vi "NIIE_Get Icon Editor Source Paths.vi"() -> (0 "IconEditorSourcePaths":path[](array[path]))   [LabVIEW 2021]
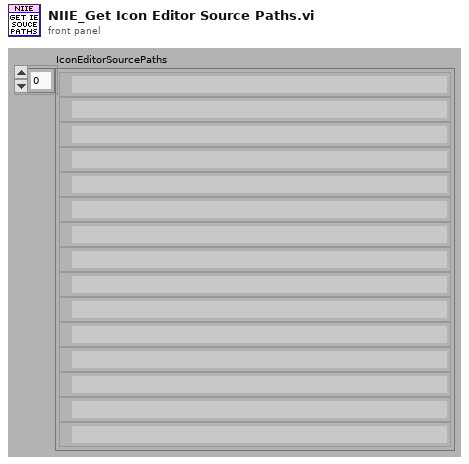
[diagram p1: front panel]
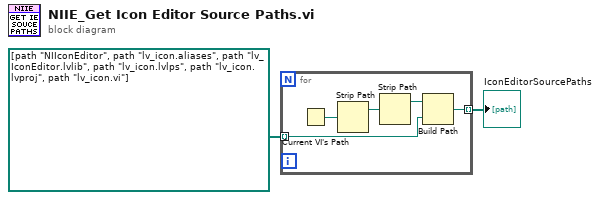
[diagram p0: block diagram]
diagram:
  n1 = for {
    tunnel: [w6] -> w2 mode=indexing
    tunnel: path[] [path "NIIconEditor", path "lv_icon.aliases", path "lv_IconEditor.lvlib", path "lv_icon.lvlps", path "lv_icon.lvproj", path "lv_icon.vi"] ("Array 2") -> [w5] mode=indexing
    n2 = Current VI's Path() -> (path=w7:path)
    n3 = Strip Path(path=w7) -> (stripped path=w4:path)  [unwired: 1 out]
    n4 = Strip Path(path=w4) -> (stripped path=w3:path)  [unwired: 1 out]
    n5 = Build Path(base path=w3, name or relative path=w5) -> (appended path=w6:path)
  }
  "IconEditorSourcePaths" <- w2
